vi "TestGitTools.vi"() -> ()   [LabVIEW 2018]
uses:
  GitCommitData.ctl
  feGEM DataPacker.lvlib
panel:
  out "Array":T1[](array[typedef])
  out ".git log paths":path[](array[path])
  out ".git hash paths":path[](array[path])
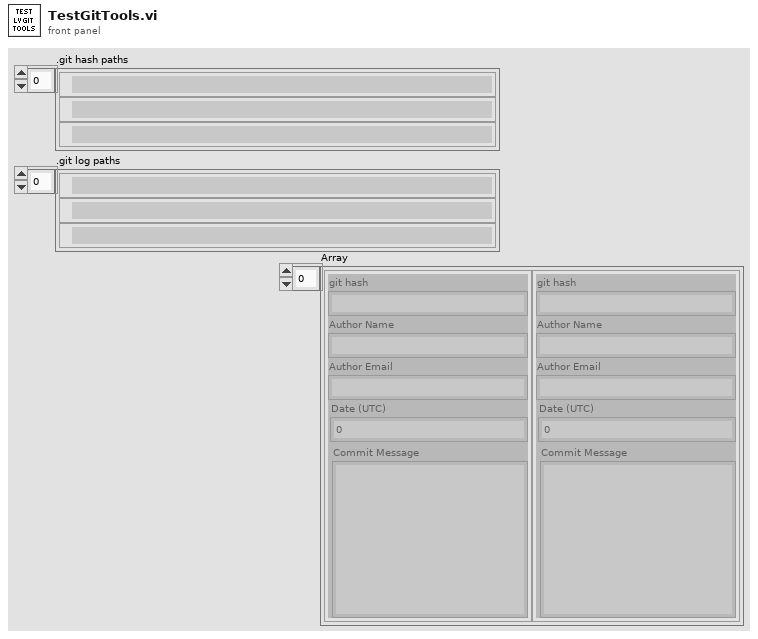
[diagram p1: front panel]
types:
  T1 = typedef "feGEM DataPacker.lvlib/GitCommitData.ctl" = cluster{"git hash":string, "Author Name":string, "Author Email":string, "Date (UTC)":i32, "Commit Message":string}
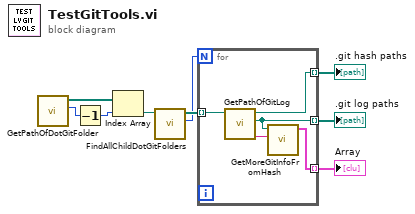
[diagram p0: block diagram]
diagram:
  n1 = call "GetPathOfDotGitFolder.vi"() -> ("Number of nested git modules"=w5:i32, ".git folder paths"=w6:path[])  [unwired: 10 in]
  n2 = Decrement(x=w5) -> (x-1=w4:i32)
  n3 = Index Array(array=w6, index=w4) -> (element=w3:path)
  n4 = call "FindAllChildDotGitFolders.vi"("Path"=w3) -> ("Number of git's including parent"=w1:i32, "All .git paths from parent"=w2:path[])  [unwired: 8 in, 1 out]
  n5 = for {
    N: w1 -> [_]
    tunnel: w2 -> [w13] mode=indexing
    tunnel: [w12] -> w9 mode=indexing
    tunnel: [w11] -> w8 mode=indexing
    tunnel: [w10] -> w7 mode=indexing
    n6 = call "GetPathOfGitLog.vi"("Path"=w13) -> ("git hash (version)"=w14:string, "git log file path"=w11:path, "git hash file path"=w12:path)  [unwired: 6 in, 2 out]
    n7 = call "GetMoreGitInfoFromHash.vi"("git hash"=w14, "git hash file path"=w11) -> ("git commit"=w10:T1)  [unwired: 8 in, 1 out]
  }
  ".git hash paths" <- w9
  ".git log paths" <- w8
  "Array" <- w7
